vi "Update Status Buffers.vi"(8 "error in (no error)":errorcluster, 11 "VeriStand DSF in":refnum<class "VeriStand DSF.lvclass">) -> (0 "error out":errorcluster, 3 "VeriStand DSF out":refnum<class "VeriStand DSF.lvclass">)   [LabVIEW 2017, in "DSF Engine.lvlib" / "VeriStand DSF.lvclass"]
uses:
  VeriStand DSF.lvclass
  DSF Core.lvlibp/Typedefs/DSF Data Type.ctl
  VeriStand DSF.lvclass/VeriStand DSF.ctl
  DSF Core.lvlibp/Classes/Buffer/Write Buffer 1D DBL.vi
  DSF Core.lvlibp/Classes/Buffer/Buffer.lvclass
  DSF Core.lvlibp/Classes/Framework/Framework.lvclass
  DSF Core.lvlibp/Classes/Framework Status/Framework Status.lvclass
  DSF Core.lvlibp
  DSF Core.lvlibp/Classes/Performance/Performance.lvclass
  C:/Git/DSF/VeriStand/Data Sharing Custom Device/Source/DSF Core.lvlibp/Classes/Framework/Framework.lvclass
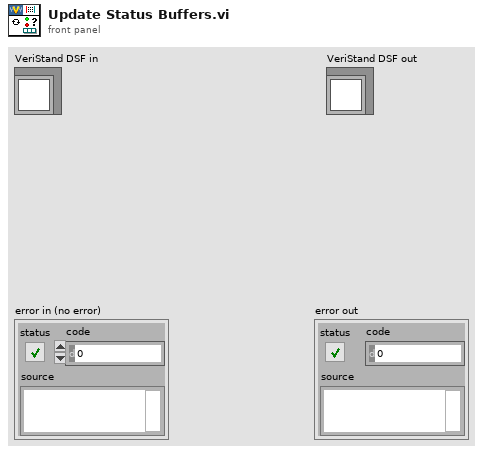
[diagram p1: front panel]
types:
  T1 = typedef "DSF Core.lvlibp/DSF Data Type.ctl" = enum8{"Bool", "SGL", "DBL", "I8", "I16", "I32", "I64", "U8", "U16", "U32", "U64"}
  T2 = typedef "DSF Core.lvlibp/Timing Status Pointer.lvclass/Timing Status Data.ctl" = cluster{"rx start time":u32, "rx end time":u32, "tx start time":u32, "tx end time":u32, "cycle start time":u32, "cycle end time":u32, "prev start time":u32}
  T3 = typedef "DSF Core.lvlibp/Status Pointer.lvclass/Status Data.ctl" = cluster{"iteration":u64, "late count":i32, "duration":u32}
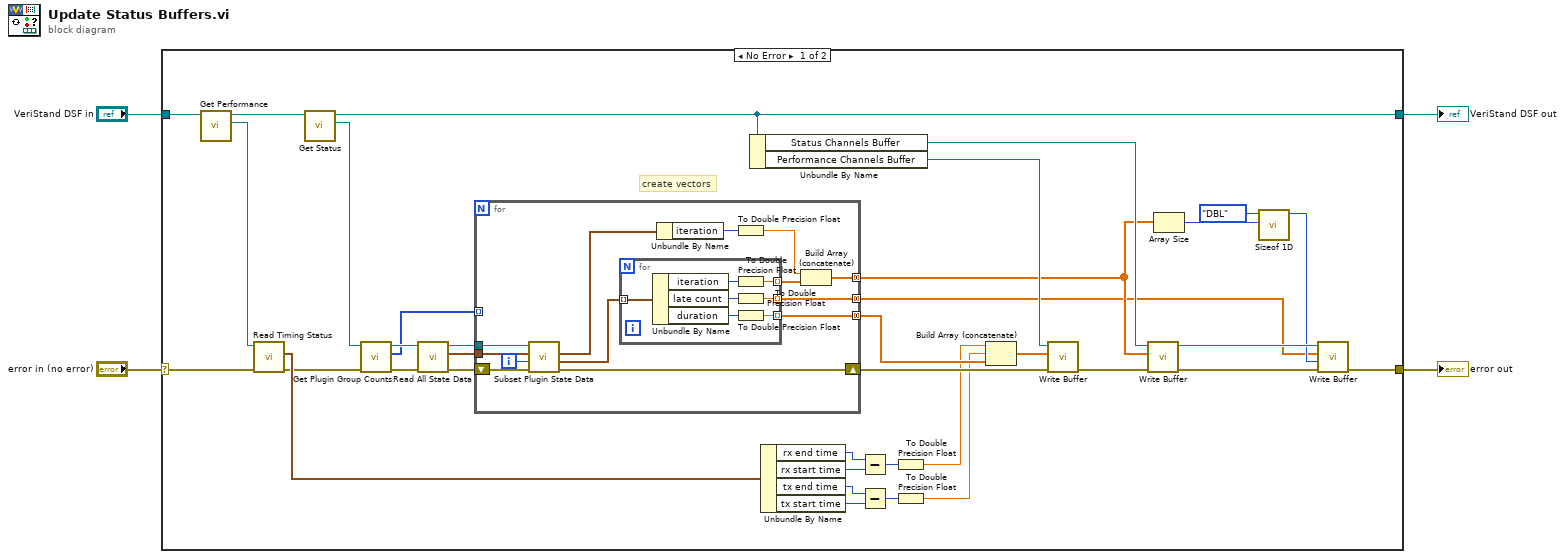
[diagram p0: block diagram]
diagram:
  n1 = case shown="No Error" "error in (no error)" {
    selector: "error in (no error)" -> [w30 w63]
    tunnel: [w36 w63] -> w3
    tunnel: "VeriStand DSF in" -> [w31 w62]
    tunnel: [w39 w62] -> w1
    frame No Error {
      # "create vectors"
      n2 = call "Get Performance.vi"("Framework in"=w31) -> ("Performance"=w28:refnum<class "Performance.lvclass">, "Framework out"=w29:refnum<class "VeriStand DSF.lvclass">)  [unwired: 9 in]
      n3 = call "Read Timing Status.vi"("error in (no error)"=w30, "Framework Performance in"=w28) -> ("error out"=w9:errorcluster, "timing status"=w27:T2)  [unwired: 7 in, 1 out]
      n4 = call "Get Status.vi"("Framework in"=w29) -> ("Status"=w8:refnum<class "Framework Status.lvclass">, "Framework out"=w39:refnum<class "VeriStand DSF.lvclass">)  [unwired: 9 in]
      n5 = call "Get Plugin Group Counts.vi"("error in (no error)"=w9, "Framework Status in"=w8) -> ("error out"=w7:errorcluster, "plugin group counts"=w5:u8[], "Framework Status out"=w6:refnum<class "Framework Status.lvclass">)  [unwired: 7 in]
      n6 = call "Read All State Data.vi"("error in (no error)"=w7, "Framework Status in"=w6) -> ("error out"=w18:errorcluster, "all state data"=w16:T3[], "Framework Status out"=w17:refnum<class "Framework Status.lvclass">)  [unwired: 7 in]
      n7 = for {
        tunnel: w17 -> [w53]
        tunnel: w16 -> [w52]
        tunnel: [w45] -> w11 mode=concatenating
        tunnel: [w44] -> w10 mode=concatenating
        tunnel: [w43] -> w15 mode=concatenating
        shift-right: [w42] -> w14
        shift-left: w18 -> [w54]
        tunnel: [w41] -> _ mode=indexing
        tunnel: w5 -> [w41] mode=indexing
        i -> [w51]
        n8 = call "Subset Plugin State Data.vi"("error in (no error)"=w54, "plugin index"=w51, "all state data"=w52, "Framework Status in"=w53) -> ("error out"=w42:errorcluster, "groups state data"=w50:T3[], "plugin state data"=w49:T3)  [unwired: 4 in, 1 out]
        n9 = for {
          tunnel: w50 -> [w61] mode=indexing
          tunnel: [w59] -> w47 mode=indexing
          tunnel: [w56] -> w44 mode=indexing
          tunnel: [w55] -> w43 mode=indexing
          n10 = Unbundle By Name(w61) -> ("iteration"=w60:u64, "late count"=w58:i32, "duration"=w57:u32)
          n11 = To Double Precision Float(number=w60) -> (double precision float=w59:dbl)
          n12 = To Double Precision Float(number=w58) -> (double precision float=w56:dbl)
          n13 = To Double Precision Float(number=w57) -> (double precision float=w55:dbl)
        }
        n14 = Unbundle By Name(w49) -> ("iteration"=w48:u64)
        n15 = To Double Precision Float(number=w48) -> (double precision float=w46:dbl)
        n16 = Build Array (concatenate)(w46, w47) -> (w45:dbl[])
      }
      n17 = Unbundle By Name(w39) -> ("Status Channels Buffer"=w34:refnum<class "Buffer.lvclass">, "Performance Channels Buffer"=w40:refnum<class "Buffer.lvclass">)
      n18 = Unbundle By Name(w27) -> ("rx end time"=w25:u32, "rx start time"=w26:u32, "tx end time"=w23:u32, "tx start time"=w24:u32)
      n19 = Subtract(x=w25, y=w26) -> (x-y=w22:u32)
      n20 = Subtract(x=w23, y=w24) -> (x-y=w21:u32)
      n21 = To Double Precision Float(number=w22) -> (double precision float=w13:dbl)
      n22 = To Double Precision Float(number=w21) -> (double precision float=w12:dbl)
      n23 = Build Array (concatenate)(w13, w12, w15) -> (w20:dbl[])
      n24 = call-poly "Write Buffer.vi"("error in (no error)"=w14, "src array in"=w20, "Buffer in"=w40) -> ("error out"=w19:errorcluster)  [unwired: 5 in, 3 out]
      n25 = call-poly "Write Buffer.vi"("error in (no error)"=w19, "src array in"=w11, "Buffer in"=w34) -> ("error out"=w35:errorcluster, "Buffer out"=w33:refnum<class "Buffer.lvclass">)  [unwired: 5 in, 2 out]
      n26 = Array Size(array=w11) -> (size(s)=w38:i32)
      n27 = call "Sizeof 1D.vi"("count"=w38, "data type"=DSF_Data_Type."DBL") -> ("size in bytes"=w32:u64)  [unwired: 9 in]
      n28 = call-poly "Write Buffer.vi"("error in (no error)"=w35, "offset (0)"=w32, "src array in"=w10, "Buffer in"=w33) -> ("error out"=w36:errorcluster)  [unwired: 4 in, 3 out]
    }
    frame Error {
    }
  }
  "error out" <- w3
  "VeriStand DSF out" <- w1
